vi "Test Timed Messaging.vi"(8 "error in":errorcluster, 11 "Test Case In":refnum<class "Messaging Tests.lvclass">) -> (0 "error out":errorcluster, 3 "Test Case Out":refnum<class "Messaging Tests.lvclass">)   [LabVIEW 2020, in "Messaging Tests.lvlib" / "Messaging Tests.lvclass"]
uses:
  Messaging Tests.lvclass
  Core/ActorFramework/Time-Delayed Send Message/Time-Delay Override Options.ctl
  Core/ActorFramework/Actor Framework.lvlib
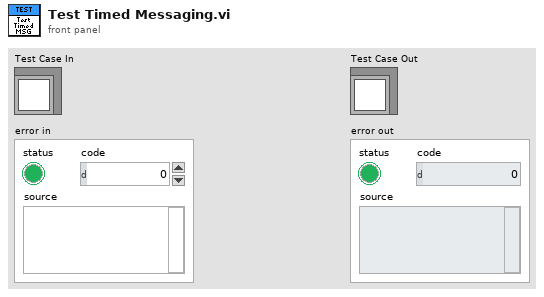
[diagram p1: front panel]
types:
  T1 = typedef "Actor Framework.lvlib/Time-Delay Override Options.ctl" = enum16{"Send next copy now", "Skip next scheduled copy", "Send next copy now and stop all further copies", "Stop all further copies"}
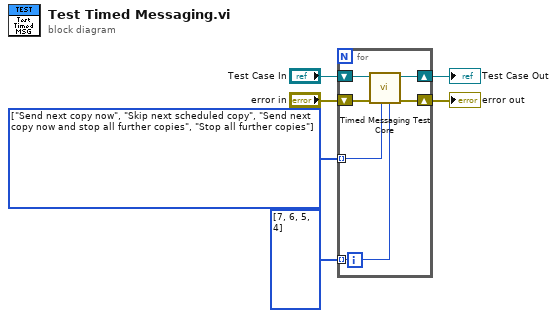
[diagram p0: block diagram]
diagram:
  w3 = T1[] [enum."Send next copy now", enum."Skip next scheduled copy", enum."Send next copy now and stop all further copies", enum."Stop all further copies"] items=["Send next copy now", "Skip next scheduled copy", "Send next copy now and stop all further copies", "Stop all further copies"]
  n1 = for {
    shift-right: [w7] -> w1
    shift-left: "Test Case In" -> [w8]
    shift-right: [w11] -> w5
    shift-left: "error in" -> [w12]
    tunnel: w3 -> [w10] mode=indexing
    tunnel: i32[] [7, 6, 5, 4] -> [w9] mode=indexing
    n2 = call "Timed Messaging Test Core.vi"("expected"=w9, "notification"=w10, "error in"=w12, "Test Case In"=w8) -> ("error out"=w11:errorcluster, "Test Case Out"=w7:refnum<class "Messaging Tests.lvclass">)  [unwired: 6 in]
  }
  "error out" <- w5
  "Test Case Out" <- w1
